vi "Adam_5056_Module.vi"(8 "Set state:":bool, 9 "Device":T2, 10 "Address (all reqd.)":T1, 11 "Channel Name":string) -> ()   [LabVIEW 2011]
uses:
  Valve_Pump.ctl
  ADAM Client/Sub VIs/ADAM Controls/Address.ctl
  Pumps_Valves_Dependencies_Global.vi
panel:
  out "Good Reply":bool
  out "Comment":string
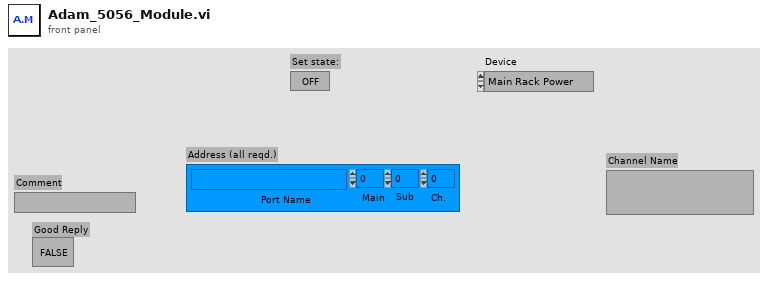
[diagram p1: front panel]
types:
  T1 = typedef "Address.ctl" = cluster{"Main":i32, "Ch.":i32, "Sub":i32, "Port Name":string}
  T2 = typedef "Valve_Pump.ctl" = enum16{"Main Rack Power", "Pump Power", "Valve Power", "V4", "V5", "V6", "V7", "V8", "V9", "V10", "V11", "V12", "V13", "V14", "V15", "V18", "V19", "V20", "V21", "V22", "V23", "V24", "V25", "V26", "V27", "V28", "V29", "V30", "V31", "V32", "V33", "V34", "Pump A", "Pump B", "Pump C", "Pump D"}
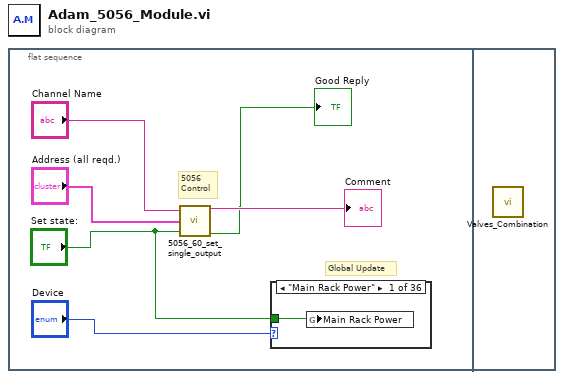
[diagram p0: block diagram]
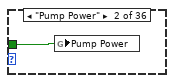
[diagram p2: hidden frame]
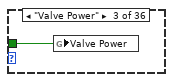
[diagram p3: hidden frame]
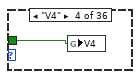
[diagram p4: hidden frame]
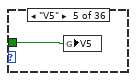
[diagram p5: hidden frame]
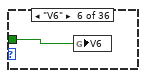
[diagram p6: hidden frame]
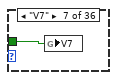
[diagram p7: hidden frame]
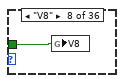
[diagram p8: hidden frame]
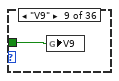
[diagram p9: hidden frame]
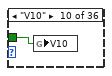
[diagram p10: hidden frame]
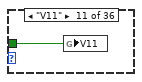
[diagram p11: hidden frame]
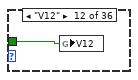
[diagram p12: hidden frame]
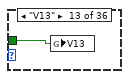
[diagram p13: hidden frame]
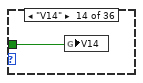
[diagram p14: hidden frame]
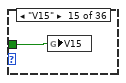
[diagram p15: hidden frame]
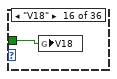
[diagram p16: hidden frame]
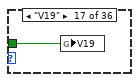
[diagram p17: hidden frame]
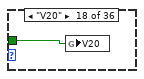
[diagram p18: hidden frame]
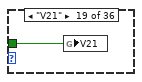
[diagram p19: hidden frame]
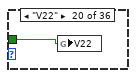
[diagram p20: hidden frame]
diagram:
  n1 = flat-sequence {
    frame #0 {
      # "5056 \nControl"
      # "Global Update"
      n2 = call "5056_60_set_single_output.vi"("Channel Name"="Channel Name", "Address (all reqd.)"="Address (all reqd.)", "Set state:"="Set state:") -> ("Comment"=→"Comment":string, "Good Reply"=→"Good Reply":bool)  [unwired: 2 in]
      n3 = case shown="\"Main Rack Power\"" "Device" {
        tunnel: "Set state:" -> [w7 w8 w9 w10 w11 w12 w13 w14 w15 w16 w17 w18 w19 w20 w21 w22 w23 w24 w25 w26 w27 w28 w29 w30 w31 w32 w33 w34 w35 w36 w37 w38 w39 w40 w41 w42]
        frame "Main Rack Power" {
          n4 = global write "Pumps_Valves_Dependencies_Global.vi" "Main Rack Power"(w7) -> ()
        }
        frame "Pump Power" {
          n5 = global write "Pumps_Valves_Dependencies_Global.vi" "Pump Power"(w8) -> ()
        }
        frame "Valve Power" {
          n6 = global write "Pumps_Valves_Dependencies_Global.vi" "Valve Power"(w9) -> ()
        }
        frame "V4" {
          n7 = global write "Pumps_Valves_Dependencies_Global.vi" "V4"(w10) -> ()
        }
        frame "V5" {
          n8 = global write "Pumps_Valves_Dependencies_Global.vi" "V5"(w11) -> ()
        }
        frame "V6" {
          n9 = global write "Pumps_Valves_Dependencies_Global.vi" "V6"(w12) -> ()
        }
        frame "V7" {
          n10 = global write "Pumps_Valves_Dependencies_Global.vi" "V7"(w13) -> ()
        }
        frame "V8" {
          n11 = global write "Pumps_Valves_Dependencies_Global.vi" "V8"(w14) -> ()
        }
        frame "V9" {
          n12 = global write "Pumps_Valves_Dependencies_Global.vi" "V9"(w15) -> ()
        }
        frame "V10" {
          n13 = global write "Pumps_Valves_Dependencies_Global.vi" "V10"(w16) -> ()
        }
        frame "V11" {
          n14 = global write "Pumps_Valves_Dependencies_Global.vi" "V11"(w17) -> ()
        }
        frame "V12" {
          n15 = global write "Pumps_Valves_Dependencies_Global.vi" "V12"(w18) -> ()
        }
        frame "V13" {
          n16 = global write "Pumps_Valves_Dependencies_Global.vi" "V13"(w19) -> ()
        }
        frame "V14" {
          n17 = global write "Pumps_Valves_Dependencies_Global.vi" "V14"(w20) -> ()
        }
        frame "V15" {
          n18 = global write "Pumps_Valves_Dependencies_Global.vi" "V15"(w21) -> ()
        }
        frame "V18" {
          n19 = global write "Pumps_Valves_Dependencies_Global.vi" "V18"(w22) -> ()
        }
        frame "V19" {
          n20 = global write "Pumps_Valves_Dependencies_Global.vi" "V19"(w23) -> ()
        }
        frame "V20" {
          n21 = global write "Pumps_Valves_Dependencies_Global.vi" "V20"(w24) -> ()
        }
        frame "V21" {
          n22 = global write "Pumps_Valves_Dependencies_Global.vi" "V21"(w25) -> ()
        }
        frame "V22" {
          n23 = global write "Pumps_Valves_Dependencies_Global.vi" "V22"(w26) -> ()
        }
        frame "V23" {
          n24 = global write "Pumps_Valves_Dependencies_Global.vi" "V23"(w27) -> ()
        }
        frame "V24" {
          n25 = global write "Pumps_Valves_Dependencies_Global.vi" "V24"(w28) -> ()
        }
        frame "V25" {
          n26 = global write "Pumps_Valves_Dependencies_Global.vi" "V25"(w29) -> ()
        }
        frame "V26" {
          n27 = global write "Pumps_Valves_Dependencies_Global.vi" "V26"(w30) -> ()
        }
        frame "V27" {
          n28 = global write "Pumps_Valves_Dependencies_Global.vi" "V27"(w31) -> ()
        }
        frame "V28" {
          n29 = global write "Pumps_Valves_Dependencies_Global.vi" "V28"(w32) -> ()
        }
        frame "V29" {
          n30 = global write "Pumps_Valves_Dependencies_Global.vi" "V29"(w33) -> ()
        }
        frame "V30" {
          n31 = global write "Pumps_Valves_Dependencies_Global.vi" "V30"(w34) -> ()
        }
        frame "V31" {
          n32 = global write "Pumps_Valves_Dependencies_Global.vi" "V31"(w35) -> ()
        }
        frame "V32" {
          n33 = global write "Pumps_Valves_Dependencies_Global.vi" "V32"(w36) -> ()
        }
        frame "V33" {
          n34 = global write "Pumps_Valves_Dependencies_Global.vi" "V33"(w37) -> ()
        }
        frame "V34" {
          n35 = global write "Pumps_Valves_Dependencies_Global.vi" "V34"(w38) -> ()
        }
        frame "Pump A" {
          n36 = global write "Pumps_Valves_Dependencies_Global.vi" "Pump A"(w39) -> ()
        }
        frame "Pump B" {
          n37 = global write "Pumps_Valves_Dependencies_Global.vi" "Pump B"(w40) -> ()
        }
        frame "Pump C" {
          n38 = global write "Pumps_Valves_Dependencies_Global.vi" "Pump C"(w41) -> ()
        }
        frame "Pump D" {
          n39 = global write "Pumps_Valves_Dependencies_Global.vi" "Pump D"(w42) -> ()
        }
      }
    }
    frame #1 {
      n40 = call "Valves_Combination.vi"() -> ()  [unwired: 12 in]
    }
  }
